vi "Init Parent.vi"(8 "error in (no error)":errorcluster, 9 "border style":i32(ring)=1 items=["None", "FixedSingle", "Fixed3D"], 10 ".net panel":refnum<k24>, 11 "[MDI] Parent in":refnum<class "[MDI] Parent.lvclass">) -> (0 "error out":errorcluster, 3 "[MDI] Parent out":refnum<class "[MDI] Parent.lvclass">)   [LabVIEW 2020, in "[MDI] Parent.lvlib" / "[MDI] Parent.lvclass"]
uses:
  [MDI] Parent.lvclass
  System.Windows.Forms
  [MDI] Parent.lvclass/[MDI] Parent.ctl
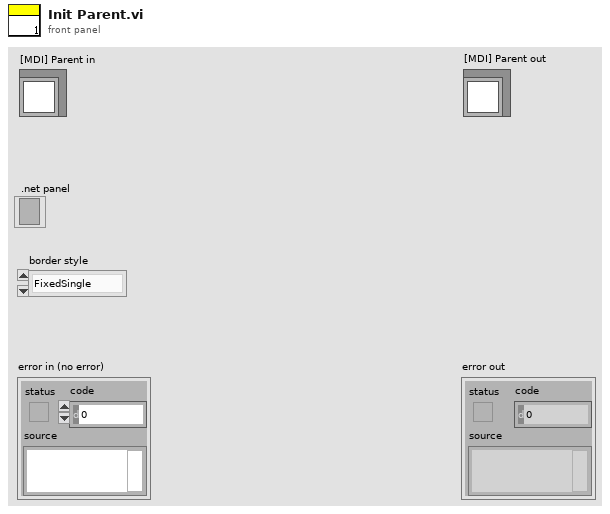
[diagram p1: front panel]
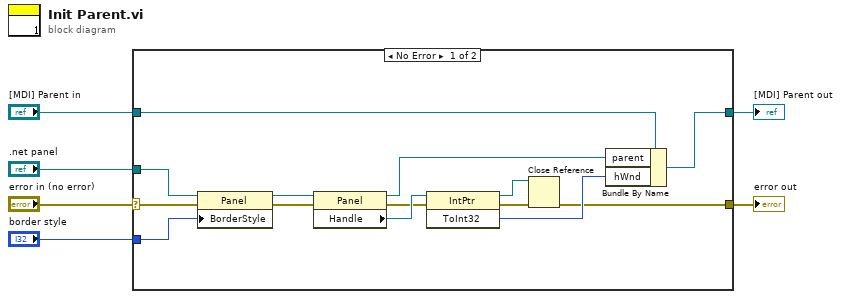
[diagram p0: block diagram]
diagram:
  n1 = case shown="No Error" "error in (no error)" {
    selector: "error in (no error)" -> [w12 w22]
    tunnel: [w9 w22] -> w5
    tunnel: [w7 w21] -> w3
    tunnel: "[MDI] Parent in" -> [w8 w21]
    tunnel: ".net panel" -> [w11 _]
    tunnel: "border style" -> [w10 _]
    frame No Error {
      n2 = property class="Panel"(reference=w11, error in=w12, "BorderStyle"=w10) -> (reference out=w17:refnum<k24>, error out=w18:errorcluster)
      n3 = property class="Panel"(reference=w17, error in=w18) -> (reference out=w14:refnum<k24>, error out=w16:errorcluster, "Handle"=w20:refnum<k24>)
      n4 = invoke class="IntPtr" method="ToInt32"(reference=w20, error in=w16) -> (reference out=w19:refnum<k24>, error out=w15:errorcluster, "ToInt32"=w13:i32)  [unwired: 1 in]
      n5 = Close Reference(reference=w19, error in (no error)=w15) -> (error out=w9:errorcluster)
      n6 = Bundle By Name(cluster=w8, "parent"=w14, "hWnd"=w13) -> (w7:refnum<class "[MDI] Parent.lvclass">)
    }
    frame Error {
    }
  }
  "error out" <- w5
  "[MDI] Parent out" <- w3
